vi "Turn T Immediatly But Ture F with Latency.vi"(7 "Reset(F)":bool, 8 "Duration(ms)":u32=5000, 11 "Signal":bool) -> (0 "Elapsed Time(ms)":u32, 3 "signal(safe)":bool)   [LabVIEW 2017]
doc: "Follows Signal, turning the output TRUE immediately but delaying the transition to FALSE by the timing duration (ms)."
uses:
  5093cefc-d3d2-4eb3-bc00-370220dfee7f.vi
  be714cb1-a87c-4b18-bbea-1129bb0f91bd.vi
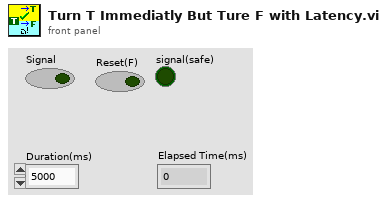
[diagram p1: front panel]
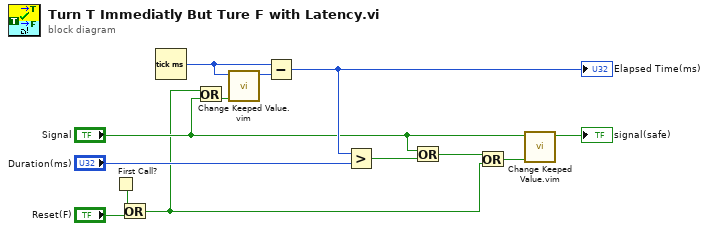
[diagram p0: block diagram]
diagram:
  n1 = First Call?() -> (First Call?: T/F=w4:bool)
  n2 = Or(x=w4, y="Reset(F)") -> (x .or. y?=w1:bool)
  n3 = Tick Count (ms)() -> (millisecond timer value=w11:u32)
  n4 = Or(x=w1, y="Signal") -> (x .or. y?=w2:bool)
  n5 = call "Change Keeped Value.vim"("change?"=w2, "new value"=w11) -> ("keeped value"=w12:u32)  [unwired: 9 in]
  n6 = Subtract(x=w11, y=w12) -> (x-y=w9:u32)
  "Elapsed Time(ms)" <- w9
  n7 = Greater?(x=w9, y="Duration(ms)") -> (0:w13:bool)
  n8 = Or(x="Signal", y=w13) -> (x .or. y?=w7:bool)
  n9 = Or(x=w7, y=w1) -> (x .or. y?=w6:bool)
  n10 = call "Change Keeped Value.vim"("change?"=w6, "new value"="Signal") -> ("keeped value"=→"signal(safe)":bool)  [unwired: 9 in]
